vi "WaitPass.vi"(10 "Target":dbl[](array[numeric]), 11 "Robot in":T1) -> (3 "Robot out":T1)   [LabVIEW 2016]
uses:
  Core/AI Robot.ctl
  Functions Enum.ctl
  AttackerStates.ctl
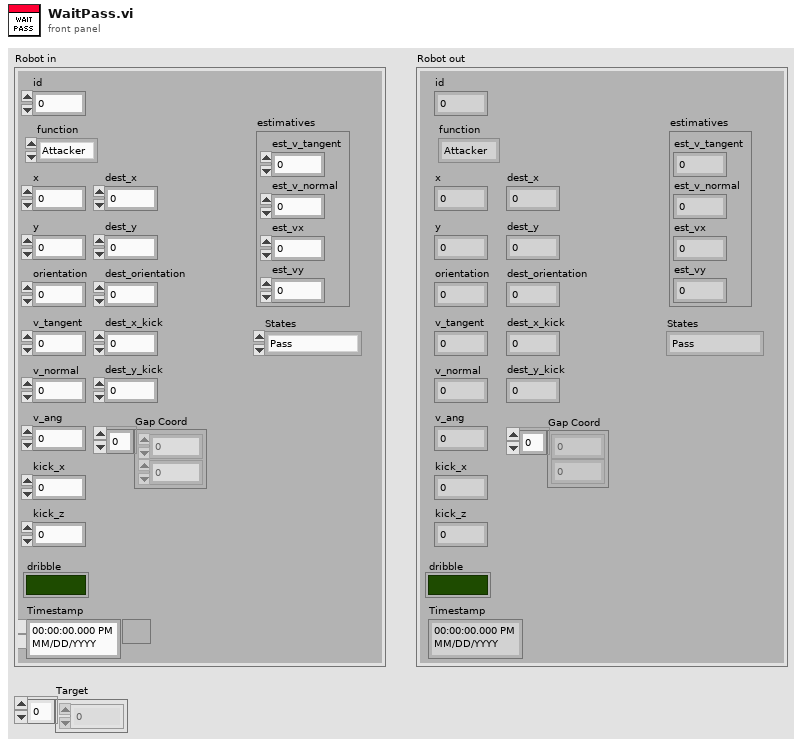
[diagram p1: front panel]
types:
  T1 = typedef "AI Robot.ctl" = cluster{"id":u32, "function":T2, "x":dbl, "y":dbl, "orientation":dbl, "v_tangent":dbl, "v_normal":dbl, "v_ang":dbl, "kick_x":dbl, "kick_z":dbl, "dribble":bool, "Timestamp":timestamp, "dest_x":dbl, "dest_y":dbl, "dest_orientation":dbl, "estimatives":cluster{"est_v_tangent":dbl, "est_v_normal":dbl, "est_vx":dbl, "est_vy":dbl}, "dest_x_kick":dbl, "dest_y_kick":dbl, "Gap Coord":dbl[], "States":T3}
  T2 = typedef "Functions Enum.ctl" = enum16{"Attacker", "Goalie", "Defender", "Striker", "Goto 0", "Dummy", "Kicker", "ZigZag"}
  T3 = typedef "AttackerStates.ctl" = enum16{"Pass", "GoToTangent", "BallGetting", "GoToKick", ""}
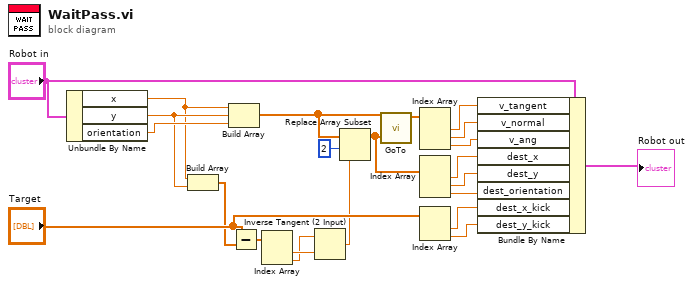
[diagram p0: block diagram]
diagram:
  n1 = Unbundle By Name("Robot in") -> ("x"=w4:dbl, "y"=w5:dbl, "orientation"=w6:dbl)
  n2 = Build Array(w4, w5) -> (w3:dbl[])
  n3 = Build Array(w4, w5, w6) -> (w13:dbl[])
  n4 = Subtract(x="Target", y=w3) -> (x-y=w7:dbl[])
  n5 = Index Array(array=w7) -> (element #1=w9:dbl, element #2=w8:dbl)  [unwired: 2 in]
  n6 = Inverse Tangent (2 Input)(1:w9, 2:w8) -> (0:w11:dbl)
  n7 = Replace Array Subset(array=w13, new element=w11, index=2) -> (w20:dbl[])
  n8 = call "GoTo.vi"("Target"=w20, "Position"=w13) -> ("Output\nVelocity"=w12:dbl[])  [unwired: 8 in, 1 out]
  n9 = Index Array(array=w12) -> (element #1=w21:dbl, element #2=w22:dbl, element #3=w23:dbl)  [unwired: 3 in]
  n10 = Index Array(array=w20) -> (element #1=w17:dbl, element #2=w18:dbl, element #3=w19:dbl)  [unwired: 3 in]
  n11 = Index Array(array="Target") -> (element #1=w15:dbl, element #2=w16:dbl)  [unwired: 2 in]
  n12 = Bundle By Name(cluster="Robot in", "v_tangent"=w21, "v_normal"=w22, "v_ang"=w23, "dest_x"=w17, "dest_y"=w18, "dest_orientation"=w19, "dest_x_kick"=w15, "dest_y_kick"=w16) -> (→"Robot out":T1)
